vi "Write Alarm Status.vi"(8 "error in":errorcluster, 10 "alarm status":T1, 11 "Value in":refnum<class "Value.lvclass">) -> (0 "error out":errorcluster, 3 "Value out":refnum<class "Value.lvclass">)   [LabVIEW 2020, in "Value.lvlib" / "Value.lvclass"]
uses:
  Value.lvclass
  Alarm Status.ctl
  Value.lvlib
  Alarm Severity.ctl
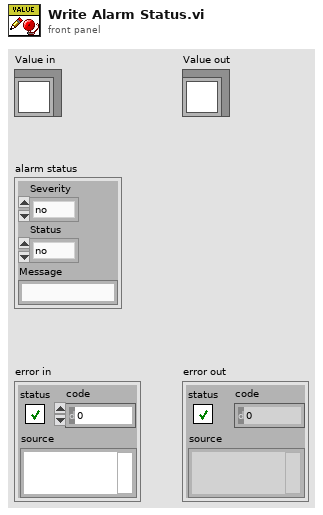
[diagram p1: front panel]
types:
  T1 = typedef "Value.lvlib/Alarm Status.ctl" = cluster{"Severity":T2, "Status":enum32{"no", "device", "driver", "record", "db", "conf", "undefined", "client"}, "Message":string}
  T2 = typedef "Value.lvlib/Alarm Severity.ctl" = enum32{"no", "minor", "major", "record", "invalid", "undefined", ""}
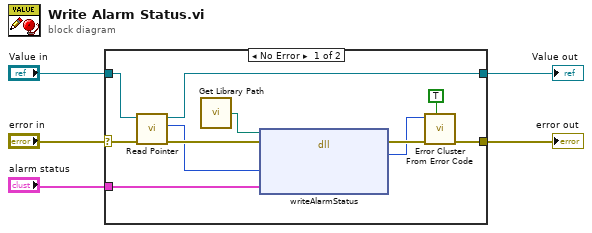
[diagram p0: block diagram]
diagram:
  n1 = case shown="No Error" "error in" {
    selector: "error in" -> [w11 w18]
    tunnel: [w12 w18] -> w5
    tunnel: "Value in" -> [w9 w17]
    tunnel: [w7 w17] -> w2
    tunnel: "alarm status" -> [w6 _]
    frame No Error {
      n2 = call-dynamic "Read Pointer.vi"("error in (no error)"=w11, "Value in"=w9) -> ("error out"=w10:errorcluster, "pointer"=w8:i64, "Value out"=w7:refnum<class "Value.lvclass">)  [unwired: 7 in]
      n3 = call "Get Library Path.vi"() -> ("Path"=w16:path)  [unwired: 1 in]
      n4 = dll-call lib="?" fn="writeAlarmStatus"(path in=w16, error in=w10, "value"=w8, "alarm status"=w6) -> (error out=w14:errorcluster, "err_code"=w13:i32)  [unwired: 3 in, 1 out]
      n5 = call <vilib>:"Error Cluster From Error Code.vi"("show call chain? (False)"=TRUE, "error in (no error)"=w14, "error code (0)"=w13) -> ("error out"=w12:errorcluster)  [unwired: 6 in]
    }
    frame Error {
    }
  }
  "error out" <- w5
  "Value out" <- w2
